vi "Teleop.vi"(10 "Match Info":T1={"Autonomous Elapsed Seconds"=0.0, "TeleOp Elapsed Seconds"=0.0, "Disabled Elapsed Seconds"=0.0, "Visited Autonomous"=FALSE, "Visited TeleOp"=FALSE, "Visited Disabled"=FALSE, "Autonomous Settings"={"Autonomous Style"=enum."Independent", "VI Refnum"=refnum}}, 11 "Call Context":T2) -> ()   [LabVIEW 2016]
doc: "This VI is called for each TeleOp packet received from the DS where the robot is not disabled. It is often used to read from the joysticks and update I/O or to update setpoints for timed control loops. It should complete and return within 20 milliseconds or it may miss DS packets."
uses:
  <vilib>/Rock Robotics/WPI/DriverStation/WPI_DriverStationDerivedRobotMode.ctl
  <vilib>/Rock Robotics/WPI/DriverStation/WPI_DriverStationMatch Info.ctl
  <vilib>/Rock Robotics/WPI/Solenoid/WPI_SolenoidValue.ctl
  <vilib>/Rock Robotics/WPI/Relay/WPI_RelayValue.ctl
  <vilib>/Rock Robotics/Network Tables/NT Read Boolean.vi
  <vilib>/Rock Robotics/Network Tables/NT Read Number.vi
  <vilib>/Rock Robotics/WPI/Utilities/WPI_GetSetVariantRefNum.vi
  <vilib>/Rock Robotics/Network Tables/NT Write Boolean Array.vi
  <vilib>/Rock Robotics/Network Tables/NT Write Numeric Array.vi
  <vilib>/Rock Robotics/WPI/Solenoid/WPI_SolenoidSetEnum.vi
  <vilib>/Rock Robotics/Network Tables/NT Write Boolean.vi
  <vilib>/Rock Robotics/WPI/RobotDrive/WPI_RobotDriveMecanumDrive_Cartesian.vi
panel:
  out "Sample Slider 0":dbl(slide) scale=0.0..5.0
  out "Sample Boolean 1":bool
  out "Sample Boolean 0":bool
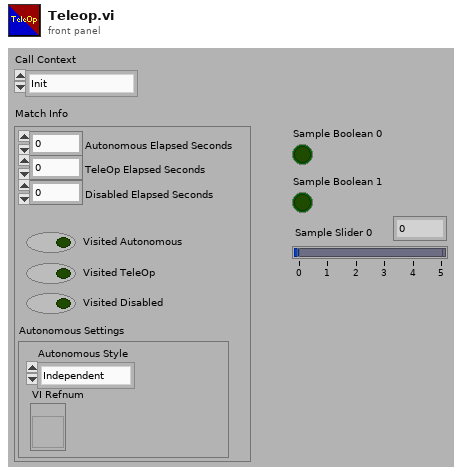
[diagram p1: front panel]
types:
  T1 = typedef "WPI_DriverStationMatch Info.ctl" = cluster{"Autonomous Elapsed Seconds":dbl, "TeleOp Elapsed Seconds":dbl, "Disabled Elapsed Seconds":dbl, "Visited Autonomous":bool, "Visited TeleOp":bool, "Visited Disabled":bool, "Autonomous Settings":cluster{"Autonomous Style":enum16{"Iterative", "Independent"}, "VI Refnum":refnum<vi>}}
  T2 = typedef "WPI_DriverStationDerivedRobotMode.ctl" = enum16{"Init", "Execute", "Stop"}
  T3 = typedef "WPI_SolenoidValue.ctl" = enum16{"Off", "On", "Forward", "Reverse"}
  T4 = typedef "WPI_MotorControlDeviceRef.ctl" = cluster{"DeviceStatus":errorcluster, "Type":T5, "PWM":cluster{"PWM Channel":T6, "DeadBand":T7}, "CAN":cluster{"Device Number":u8, "SetOutput VI Ref":variant, "GetOutput VI Ref":variant, "Enable VI Ref":variant, "Disable VI Ref":variant, "Data":variant}, "Invert":bool}
  T5 = typedef "WPI_MotorControlType.ctl" = enum16{"PWM", "CAN"}
  T6 = typedef "FPGA_DIOPWMChannel.ctl" = enum8{"PWM 0", "PWM 1", "PWM 2", "PWM 3", "PWM 4", "PWM 5", "PWM 6", "PWM 7", "PWM 8", "PWM 9", "PWM MXP 0", "PWM MXP 1", "PWM MXP 2", "PWM MXP 3", "PWM MXP 4", "PWM MXP 5", "PWM MXP 6", "PWM MXP 7", "PWM MXP 8", "PWM MXP 9", "Invalid"}
  T7 = typedef "WPI_PWMDeadband.ctl" = cluster{"Name":string, "maxPositivePwm":i32, "minPositivePwm":i32, "centerPwm":i32, "maxNegativePwm":i32, "minNegativePwm":i32, "angularRange":u16}
  T8 = typedef "WPI_JoystickDevRef.ctl" = cluster{"Device":T9}
  T9 = typedef "WPI_JoystickDeviceEnum.ctl" = enum16{"USB 0", "USB 1", "USB 2", "USB 3", "USB 4", "USB 5"}
  T10 = typedef "WPI_SolenoidDevRef.ctl" = cluster{"DevStatus":errorcluster, "Pneumatics Control Module":u8, "Forward Solenoid Channel":T11, "Reverse Solenoid Channel":T11}
  T11 = typedef "WPI_SolenoidChannel.ctl" = enum8{"Solenoid 0", "Solenoid 1", "Solenoid 2", "Solenoid 3", "Solenoid 4", "Solenoid 5", "Solenoid 6", "Solenoid 7", "Invalid"}
  T12 = typedef "WPI_RobotDriveDevRef.ctl" = cluster{"DevStatus":errorcluster, "Motors[]":T4[], "Square Inputs":bool, "Max Output":dbl}
  T13 = typedef "WPI_CompressorDevRef.ctl" = cluster{"DevStatus":errorcluster, "Pneumatics Control Module":u8}
  T14 = typedef "WPI_RelayValue.ctl" = enum16{"Off", "On", "Forward", "Reverse"}
  T15 = typedef "WPI_RelayDevRef.ctl" = cluster{"DevStatus":errorcluster, "Relay Channel":T16, "Relay Direction":T17}
  T16 = typedef "FPGA_DIORelayChannel.ctl" = enum8{"Relay 0", "Relay 1", "Relay 2", "Relay 3", "Invalid"}
  T17 = typedef "WPI_RelayDirection.ctl" = enum16{"Both directions", "Forward only", "Reverse only"}
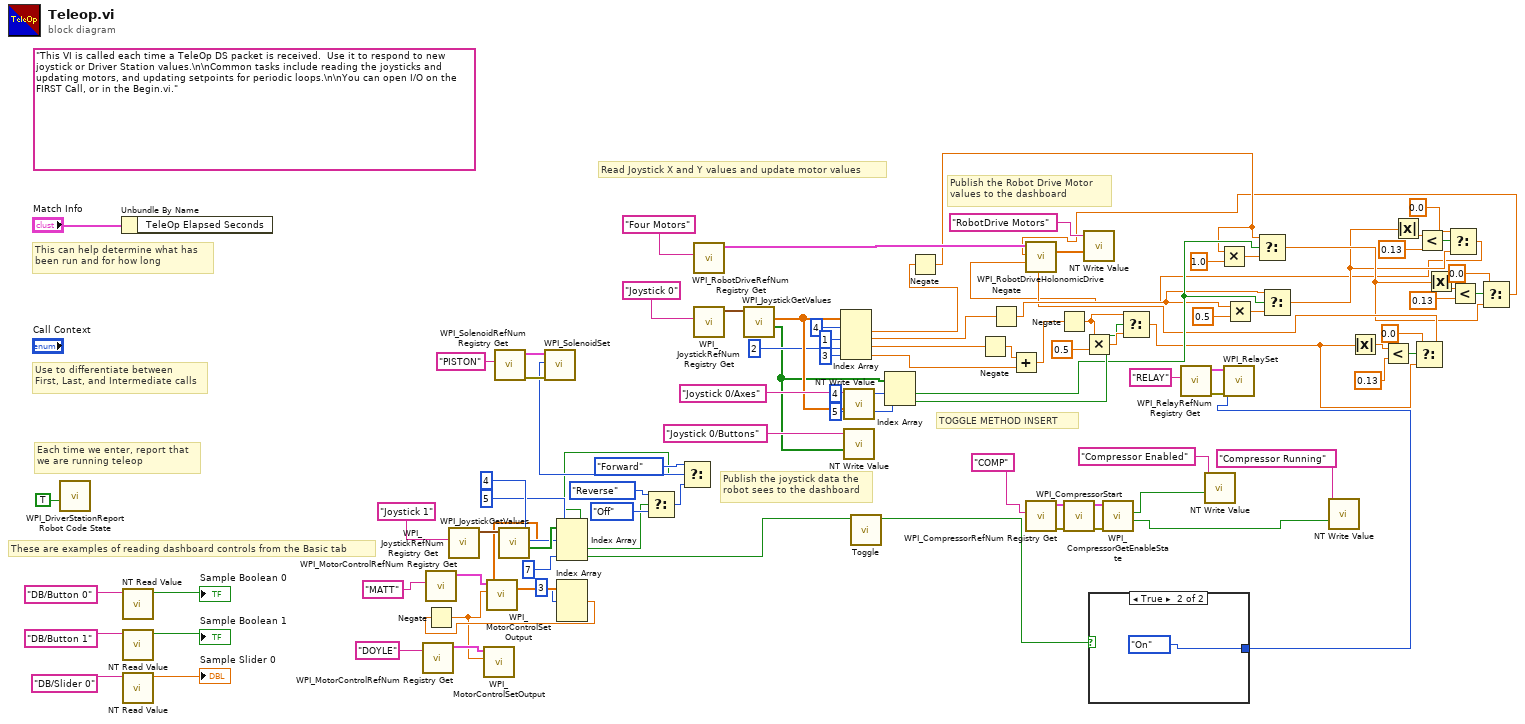
[diagram p0: block diagram]
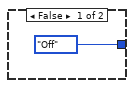
[diagram p2: hidden frame]
diagram:
  (unwired) "This VI is called each time a TeleOp DS packet is received.  Use it to respond to new joystick or Driver Station values.\n\nCommon tasks include reading the joysticks and updating motors, and updating setpoints for periodic loops.\n\nYou can open I/O on the FIRST Call, or in the Begin.vi."
  # "TOGGLE METHOD INSERT"
  # "Publish the Robot Drive Motor\nvalues to the dashboard"
  # "Publish the joystick data the\nrobot sees to the dashboard"
  # "Read Joystick X and Y values and update motor values"
  # "These are examples of reading dashboard controls from the Basic tab"
  # "Each time we enter, report that\nwe are running teleop"
  # "Use to differentiate between\nFirst, Last, and Intermediate calls"
  # "This can help determine what has\nbeen run and for how long"
  n1 = call <vilib>:"WPI_DriverStationReport Robot Code State.vi"("TeleOp"=TRUE ("Autonomous")) -> ()  [unwired: 10 in, 1 out]
  n2 = Unbundle By Name("Match Info") -> ()  [unwired: 1 out]
  n3 = call-poly <vilib>:"NT Read Value.vi"("Name"="DB/Button 0" ("refnum name")) -> ("Boolean"=→"Sample Boolean 0":bool)  [unwired: 9 in, 1 out]
  n4 = call-poly <vilib>:"NT Read Value.vi"("Name"="DB/Button 1" ("refnum name")) -> ("Boolean"=→"Sample Boolean 1":bool)  [unwired: 9 in, 1 out]
  n5 = call-poly <vilib>:"NT Read Value.vi"("Name"="DB/Slider 0" ("refnum name")) -> ("Numeric"=→"Sample Slider 0":dbl)  [unwired: 9 in, 1 out]
  n6 = call <vilib>:"WPI_MotorControlRefNum Registry Get.vi"("refnum name"="DOYLE") -> ("MotorControlDevRef"=w54:T4)  [unwired: 9 in, 1 out]
  n7 = call <vilib>:"WPI_MotorControlRefNum Registry Get.vi"("refnum name"="MATT") -> ("MotorControlDevRef"=w53:T4)  [unwired: 9 in, 1 out]
  n8 = call <vilib>:"WPI_JoystickRefNum Registry Get.vi"("refnum name"="Joystick 1") -> ("JoystickDevRef"=w70:T8)  [unwired: 1 in, 9 out]
  n9 = call <vilib>:"WPI_SolenoidRefNum Registry Get.vi"("refnum name"="PISTON") -> ("error out"=w65:errorcluster, "SolenoidDevRef"=w64:T10)  [unwired: 9 in]
  n10 = call <vilib>:"WPI_JoystickGetValues.vi"("JoystickDevRef"=w70) -> ("Buttons"=w69:bool[], "Axes"=w52:dbl[])  [unwired: 6 in, 3 out]
  n11 = Index Array(array=w69, index #1=4 ("index"), index #2=5 ("index"), index #3=7 ("index")) -> (element #1=w58:bool, element #2=w57:bool, element #3=w42:bool)
  n12 = Index Array(array=w52, index #1=3 ("index")) -> (element #1=w50:dbl)  [unwired: 2 in, 2 out]
  n13 = Negate(x=w50) -> (-x=w49:dbl)
  n14 = call <vilib>:"WPI_MotorControlSetOutput.vi"("Output"=w49, "MotorControlDevRef"=w54) -> ()  [unwired: 7 in, 3 out]
  n15 = call <vilib>:"WPI_MotorControlSetOutput.vi"("Output"=w49, "MotorControlDevRef"=w53) -> ()  [unwired: 7 in, 3 out]
  n16 = Select(t=WPI_SolenoidValue."Reverse" ("Value"), s=w57, f=WPI_SolenoidValue."Off" ("Value")) -> (s? t:f=w61:T3)
  n17 = Select(t=WPI_SolenoidValue."Forward" ("Value"), s=w58, f=w61) -> (s? t:f=w63:T3)
  n18 = call-poly <vilib>:"WPI_SolenoidSet.vi"("error in (no error)"=w65, "Value"=w63, "SolenoidDevRef"=w64) -> ()  [unwired: 7 in, 2 out]
  n19 = call <vilib>:"WPI_RobotDriveRefNum Registry Get.vi"("refnum name"="Four Motors") -> ("RobotDriveDevRef"=w89:T12)  [unwired: 1 in, 9 out]
  n20 = call <vilib>:"WPI_JoystickRefNum Registry Get.vi"("refnum name"="Joystick 0") -> ("JoystickDevRef"=w87:T8)  [unwired: 1 in, 9 out]
  n21 = call <vilib>:"WPI_JoystickGetValues.vi"("JoystickDevRef"=w87) -> ("Buttons"=w32:bool[], "Axes"=w85:dbl[])  [unwired: 6 in, 3 out]
  n22 = Index Array(array=w85, index #1=4 ("index"), index #2=1 ("index"), index #3=2 ("index"), index #4=3 ("index")) -> (element #1=w80:dbl, element #2=w81:dbl, element #3=w75:dbl, element #4=w73:dbl)
  n23 = call-poly <vilib>:"NT Write Value.vi"("Numeric Array"=w85, "Name"="Joystick 0/Axes") -> ()  [unwired: 9 in, 1 out]
  n24 = call-poly <vilib>:"NT Write Value.vi"("Boolean Array"=w32, "Name"="Joystick 0/Buttons") -> ()  [unwired: 9 in, 1 out]
  n25 = call "Toggle.vi"("Button Input"=w42) -> ("Toggle Output"=w37:bool)  [unwired: 9 in, 1 out]
  n26 = Index Array(array=w32, index #1=4 ("index"), index #2=5 ("index")) -> (element #1=w23:bool, element #2=w24:bool)
  n27 = Negate(x=w80) -> (-x=w22:dbl)
  n28 = Negate(x=w75) -> (-x=w74:dbl)
  n29 = Negate(x=w81) -> (-x=w19:dbl)
  n30 = Add(x=w74, y=w73) -> (x+y=w72:dbl)
  n31 = call <vilib>:"WPI_CompressorRefNum Registry Get.vi"("refnum name"="COMP") -> ("error out"=w47:errorcluster, "CompressorDevRef"=w46:T13)  [unwired: 9 in]
  n32 = Negate(x=w72) -> (-x=w27:dbl)
  n33 = call <vilib>:"WPI_CompressorStart.vi"("error in (no error)"=w47, "CompressorDevRef"=w46) -> ("error out"=w45:errorcluster, "CompressorDevRef"=w44:T13)  [unwired: 8 in]
  n34 = Multiply(x=w27, y=0.5) -> (x*y=w28:dbl)
  n35 = case shown="True" w37 {
    tunnel: [WPI_RelayValue."Off" ("RelayValue") WPI_RelayValue."On" ("RelayValue")] -> w33
    frame False {
    }
    frame True {
    }
  }
  n36 = call <vilib>:"WPI_CompressorGetEnableState.vi"("error in (no error)"=w45, "CompressorDevRef"=w44) -> ("Compressor Running"=w38:bool, "Enabled"=w39:bool)  [unwired: 6 in, 2 out]
  n37 = Select(t=w27, s=w24, f=w28) -> (s? t:f=w6:dbl)
  n38 = call <vilib>:"WPI_RelayRefNum Registry Get.vi"("refnum name"="RELAY") -> ("error out"=w35:errorcluster, "RelayDevRef"=w34:T15)  [unwired: 9 in]
  n39 = call-poly <vilib>:"NT Write Value.vi"("Boolean"=w39, "Name"="Compressor Enabled") -> ()  [unwired: 9 in, 1 out]
  n40 = Multiply(x=w22, y=1.0) -> (x*y=w29:dbl)
  n41 = call <vilib>:"WPI_RelaySet.vi"("error in (no error)"=w35, "RelayValue"=w33, "RelayDevRef"=w34) -> ()  [unwired: 7 in, 2 out]
  n42 = Multiply(x=w19, y=0.5) -> (x*y=w25:dbl)
  n43 = Select(t=w22, s=w23, f=w29) -> (s? t:f=w4:dbl)
  n44 = Select(t=w19, s=w23, f=w25) -> (s? t:f=w2:dbl)
  n45 = call-poly <vilib>:"NT Write Value.vi"("Boolean"=w38, "Name"="Compressor Running") -> ()  [unwired: 9 in, 1 out]
  n46 = Absolute Value(x=w6) -> (abs(x)=w15:dbl)
  n47 = Less?(x=w15, y=0.13) -> (x < y?=w18:bool)
  n48 = Absolute Value(x=w2) -> (abs(x)=w11:dbl)
  n49 = Select(t=0.0, s=w18, f=w6) -> (s? t:f=w5:dbl)
  n50 = Less?(x=w11, y=0.13) -> (x < y?=w16:bool)
  n51 = Absolute Value(x=w4) -> (abs(x)=w10:dbl)
  n52 = Select(t=0.0, s=w16, f=w2) -> (s? t:f=w1:dbl)
  n53 = Less?(x=w10, y=0.13) -> (x < y?=w17:bool)
  n54 = Select(t=0.0, s=w17, f=w4) -> (s? t:f=w3:dbl)
  n55 = call-poly <vilib>:"WPI_RobotDriveHolonomicDrive.vi"("Rotation"=w5, "Y"=w1, "X"=w3, "RobotDriveDevRef"=w89) -> ("Motor Values"=w83:dbl[])  [unwired: 5 in, 2 out]
  n56 = call-poly <vilib>:"NT Write Value.vi"("Numeric Array"=w83, "Name"="RobotDrive Motors") -> ()  [unwired: 9 in, 1 out]
